vi "Calculate Triangle Illumination.vi"(6 "Fill Colour":u32(colorbox)=12517256, 7 "Light Direction":T1, 11 "Triangle Normal":T1) -> (3 "Fill Colour Actual":u32(colorbox)=12517256)   [LabVIEW 2020, in "3D (FPGA).lvlib"]
uses:
  3D (FPGA).lvlib
  Vector 3D.ctl
panel:
  in  "y":sgl=0.01
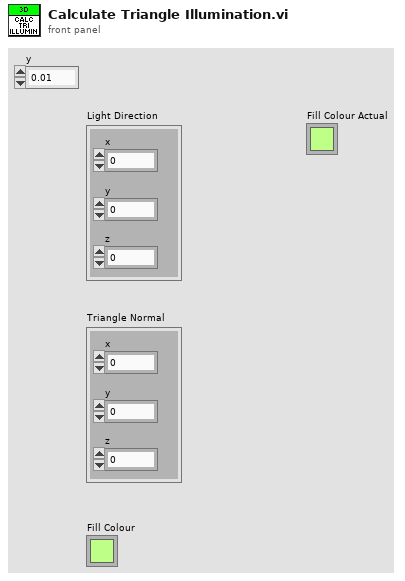
[diagram p1: front panel]
types:
  T1 = typedef "3D (FPGA).lvlib/Vector 3D.ctl" = cluster{"x":sgl, "y":sgl, "z":sgl}
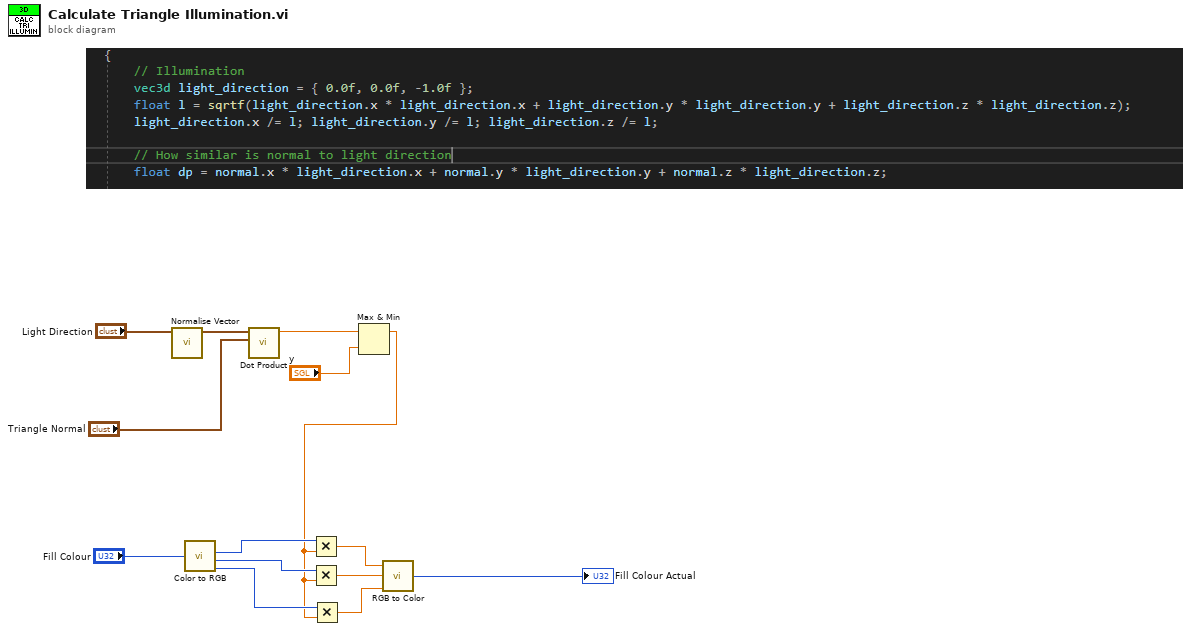
[diagram p0: block diagram]
diagram:
  n1 = call "Normalise Vector.vi"("Vector 3D"="Light Direction") -> ("Vector 3D Normalised"=w13:T1)  [unwired: 10 in]
  n2 = call <vilib>:"Color to RGB.vi"("Color"="Fill Colour") -> ("R"=w9:u8, "G"=w10:u8, "B"=w8:u8)  [unwired: 1 out]
  n3 = call "Dot Product.vi"("Vector B"="Triangle Normal", "Vector A"=w13) -> ("Dot Product"=w2:sgl)  [unwired: 9 in]
  n4 = Max & Min(x=w2, y="y") -> (max(x,y)=w1:sgl)  [unwired: 1 out]
  n5 = Multiply(x=w9, y=w1) -> (x*y=w7:sgl)
  n6 = Multiply(x=w10, y=w1) -> (x*y=w6:sgl)
  n7 = Multiply(x=w8, y=w1) -> (x*y=w5:sgl)
  n8 = call <vilib>:"RGB to Color.vi"("B"=w5, "G"=w6, "R"=w7) -> ("Color"=→"Fill Colour Actual":u32)
